vi "Core.vi"(11 "Instr in":refnum<class "Instrument.lvclass">) -> ()   [LabVIEW 2016, in "Instrument.lvclass"]
uses:
  Instrument.lvclass
  Instrument.lvclass/Instrument.ctl
  Read Data OK_.vi
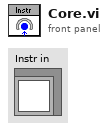
[diagram p1: front panel]
types:
  T1 = typedef "Instrument.lvclass/state.ctl" = enum8{"Configure", "Acquire", "Wait", "Quit", "Handle Error", "NOOP"}
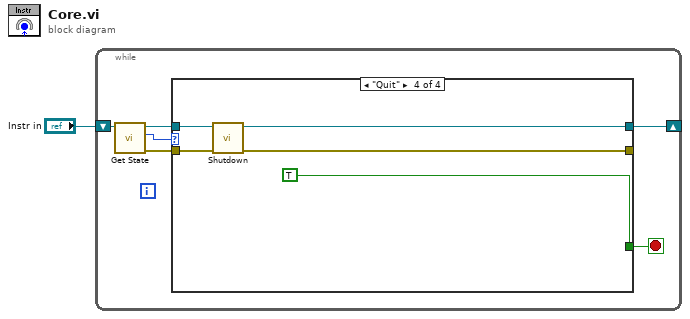
[diagram p0: block diagram]
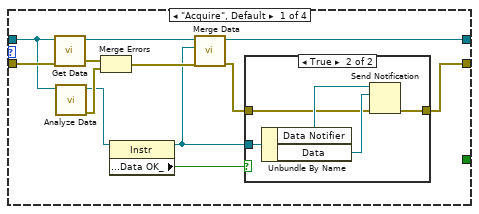
[diagram p2: hidden frame]
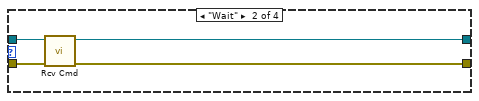
[diagram p4: hidden frame]
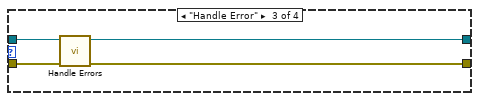
[diagram p5: hidden frame]
diagram:
  n1 = while "Acquisition" {
    shift-right: [w2] -> _
    shift-left: "Instr in" -> [w6]
    stop <- w3 stop-if-true
    n2 = call "Get State.vi"("Instrument in"=w6) -> ("error out"=w4:errorcluster, "default state"=w7:T1, "Instrument out"=w5:refnum<class "Instrument.lvclass">)  [unwired: 8 in]
    n3 = case shown="\"Quit\"" w7 {
      tunnel: w5 -> [w18 w29 w33 w37]
      tunnel: w4 -> [w19 w28 w32 w36]
      tunnel: [_ _ _ TRUE] -> w3
      tunnel: [w14 w27 w30 w35] -> w2
      tunnel: [w11 w26 w31 w34] -> _
      frame "Acquire", Default {
        n4 = call-dynamic "Get Data.vi"("error in"=w19, "Instrument in"=w18) -> ("error out"=w17:errorcluster, "Instrument out"=w15:refnum<class "Instrument.lvclass">)  [unwired: 8 in]
        n5 = call-dynamic "Analyze Data.vi"("Instrument in"=w18) -> ("error out"=w16:errorcluster, "Instrument out"=w10:refnum<class "Instrument.lvclass">)  [unwired: 9 in]
        n6 = Merge Errors(w17, w16) -> (w13:errorcluster)
        n7 = property class="Instr"(reference=w10) -> (reference out=w8:refnum<class "Instrument.lvclass">, "Accessors:Data OK_"=w9:bool)  [unwired: 1 in, 1 out]
        n8 = call-dynamic "Merge Data.vi"("error in"=w13, "Analyzed"=w8, "Acquired"=w15) -> ("error out"=w12:errorcluster, "Instrument out"=w14:refnum<class "Instrument.lvclass">)  [unwired: 7 in]
        n9 = case shown="True" w9 {
          tunnel: w8 -> [_ w25]
          tunnel: w12 -> [w20 w22]
          tunnel: [w20 w21] -> w11
          frame False {
          }
          frame True {
            n10 = Unbundle By Name(w25) -> ("Data Notifier"=w24:refnum<notifier>, "Data"=w23:refnum<class "Data.lvclass">)
            n11 = Send Notification(notification=w23, notifier=w24, error in (no error)=w22) -> (error out=w21:errorcluster)  [unwired: 1 out]
          }
        }
      }
      frame "Wait" {
        n12 = call-dynamic "Rcv Cmd.vi"("error in"=w28, "Instrument in"=w29) -> ("error out"=w26:errorcluster, "Instrument out"=w27:refnum<class "Instrument.lvclass">)  [unwired: 8 in]
      }
      frame "Handle Error" {
        n13 = call-dynamic "Handle Errors.vi"("error in"=w32, "Instrument in"=w33) -> ("error out"=w31:errorcluster, "Instrument out"=w30:refnum<class "Instrument.lvclass">)  [unwired: 7 in, 1 out]
      }
      frame "Quit" {
        n14 = call-dynamic "Shutdown.vi"("error in"=w36, "Instrument in"=w37) -> ("error out"=w34:errorcluster, "Instrument out"=w35:refnum<class "Instrument.lvclass">)  [unwired: 8 in]
      }
    }
  }
